vi "GMLAN ReadDataByPacketIdentifier.vi"(8 "error in (no error)":errorcluster, 9 "DPIDs":u8[](array[numeric]), 10 "Sub Function":T3, 11 "diag ref in":T1) -> (0 "error out":errorcluster, 1 "success?":bool, 2 "data out":u8[](array[numeric]), 3 "diag ref out":T1)   [LabVIEW 2015, in "GMLAN.lvlib"]
uses:
  GMLAN.lvlib
  _SubVIs/ReadDataByPacketIdentifier_SubFunctions.ctl
  <vilib>/Automotive Diagnostic Command Set/Diagnostic Transport.llb/Diag Reference.ctl
  <vilib>/Automotive Diagnostic Command Set/Diagnostic Transport.llb/Transport Protocol Selector.ctl
  <vilib>/Automotive Diagnostic Command Set/Diagnostic Transport.llb/Diag CAN Frame Log.ctl
  <vilib>/addons/Automotive Diagnostic Command Set/NI_Automotive Diagnostic Command Set.lvlib
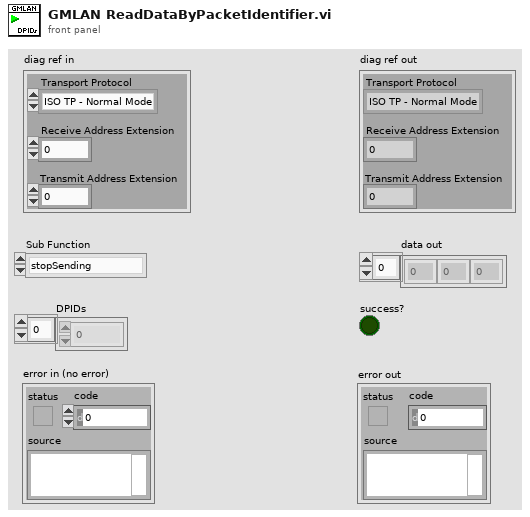
[diagram p1: front panel]
types:
  T1 = typedef "NI_Automotive Diagnostic Command Set.lvlib/Diag Reference.ctl" = cluster{"Diag CAN Handle":u32, "Transport Protocol":T2, "Receive Address Extension":u8, "Transmit Address Extension":u8, "Receive CAN Id":u32, "Transmit CAN Id":u32, "Diag CAN Queue":refnum<queue>, "Log Frames ?":bool, "My TP Address":u8, "Other TP Address":u8, "T1":u16, "T2":u16, "T3":u16, "T4":u16, "Tx SN":u8, "Block Size":u8, "Rx SN":u8, "VW TP Initialized?":bool, "Tx block no":u8, "baud rate":u32, "Interface":string, "Channel Diag CAN Handle":u32, "UDP Connection ID":refnum<k16>, "TCP Connection ID":refnum<k5>, "Target IP Addr":u32, "Source Address":u16, "Target Address":u16, "Send Header NACK?":bool, "DLL Handle":u32, "NAD":u8, "Time Stamp read first":dbl, "Time Stamp read last":dbl, "Time Stamp write first":dbl, "Time Stamp write last":dbl, "Time Stamp write":dbl, "Time Stamp read":dbl}
  T2 = typedef "NI_Automotive Diagnostic Command Set.lvlib/Transport Protocol Selector.ctl" = enum16{"ISO TP - Normal Mode", "ISO TP - Mixed Mode", "VW TP 2.0", "Diagnostics on IP", "ISO TP LIN"}
  T3 = typedef "GMLAN.lvlib/ReadDataByPacketIdentifier_SubFunctions.ctl" = enum8{"stopSending", "sendOneResponse", "scheduleAtSlowRate", "scheduleAtMediumRate", "scheduleAtFastRate"}
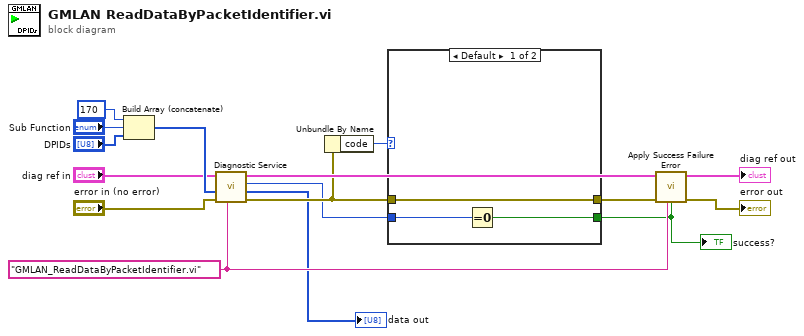
[diagram p0: block diagram]
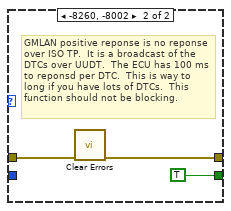
[diagram p2: hidden frame]
diagram:
  w8 = "GMLAN_ReadDataByPacketIdentifier.vi" ("error source")
  n1 = Build Array (concatenate)(u8 170 ("element"), "Sub Function", "DPIDs") -> (w12:u8[])
  n2 = call <vilib>:"Diagnostic Service.vi"("error source"=w8, "error in (no error)"="error in (no error)", "data in"=w12, "diag ref in"="diag ref in") -> ("error out"=w13:errorcluster, "data out"=→"data out":u8[], "error code"=w1:u8, "diag ref out"=→"diag ref out":T1)  [unwired: 2 in, 2 out]
  n3 = Unbundle By Name(w13) -> ("code"=w7:i32)
  n4 = case shown="Default" w7 {
    tunnel: w13 -> [w18 w21]
    tunnel: [w18 w20] -> w6
    tunnel: [w16 TRUE] -> w2
    tunnel: w1 -> [w17 _]
    frame Default {
      n5 = Equal To 0?(x=w17) -> (x = 0?=w16:bool)
    }
    frame -8260, -8002 {
      # "GMLAN positive reponse is no reponse over ISO TP.  It is a broadcast of the DTCs over UUDT.  The ECU has 100 ms to reponsd per DTC.  This is way to long if you have lots of DTCs.  This function should not be blocking."
      n6 = call <vilib>:"Clear Errors.vi"("error in (no error)"=w21) -> ("error out"=w20:errorcluster)  [unwired: 5 in, 1 out]
    }
  }
  "success?" <- w2
  n7 = call <vilib>:"Apply Success Failure Error.vi"("success code"=w2, "error source"=w8, "error in (no error)"=w6) -> ("error out"=→"error out":errorcluster)  [unwired: 8 out]
